vi "exercice6-3.vi"() -> ()   [LabVIEW 2013]
panel:
  out "Graphe":dbl[](graph)
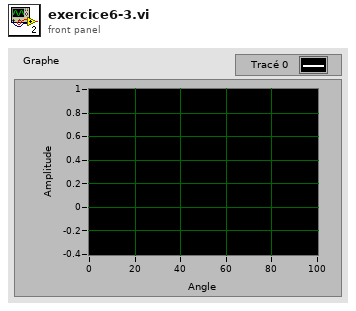
[diagram p1: front panel]
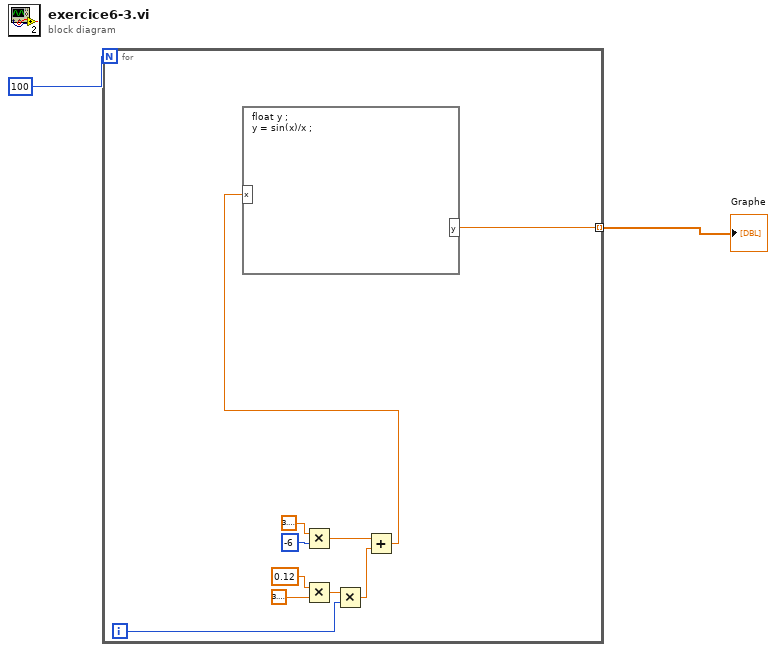
[diagram p0: block diagram]
diagram:
  n1 = for {
    N: 100 -> [_]
    tunnel: [w3] -> w1 mode=indexing
    i -> [w7]
    n2 = Multiply(x=3.141592653589793, y=-6) -> (x*y=w5:dbl)
    n3 = Multiply(x=0.12, y=3.141592653589793) -> (x*y=w8:dbl)
    n4 = Multiply(x=w8, y=w7) -> (x*y=w6:dbl)
    n5 = Add(x=w5, y=w6) -> (x+y=w4:dbl)
    n6 = formula code="float y ;\ny = sin(x)/x ;"("x"=w4) -> ("y"=w3:dbl)
  }
  "Graphe" <- w1
